vi "PH_PPPA_PowerUnit.PS Close RR.vi"(0 "i ref in":refnum<vi>, 5 "error in (no error)":errorcluster) -> (14 "i ref out":refnum<vi>, 19 "error out":errorcluster)   [LabVIEW 2014, in "PH_PPPA_PowerUnit.lvlib"]
uses:
  PH_PPPA_PowerUnit.lvlib
  PH_Beckhoff_PP_PU/PH_Beckhoff_PP_PU.lvlib
  PH_PowerUnit_BaseClass/PH_PowerUnit_BaseClass.lvlib
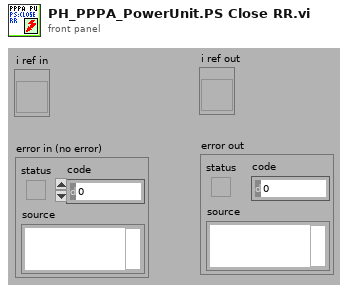
[diagram p1: front panel]
types:
  T1 = typedef "PH_PPPA_PowerUnit.lvlib/PH_PPPA_PowerUnit.i attribute.ctl" = cluster{"GUI Refs":cluster{"Ignitron":refnum<vi>, "Rossrelais":refnum<vi>, "Set Voltage":refnum<vi>, "PSU":refnum<vi>, "EOC":refnum<vi>, "Trigger":refnum<vi>}, "Ignitron":T2, "PSU":T4, "Dump Ross Relais":T5, "Trigger":cluster{"State Device":T3, "linked?":bool}, "Timing Settings":cluster{"Prdc Fast?":bool, "Default Value Periodic Interval":i32, "Mercury on since":dbl, "Warm up Time Mercury [s]":dbl}, "Set Voltage [V]":dbl, "19er Ignitionbox":string}
  T2 = typedef "PH_PP_Common.lvlib/PH_PP_Common.Ignitron Attributes.ctl" = cluster{"State Device":T3, "linked?":bool}
  T3 = typedef "PH_StatusHandler.lvlib/PH_StatusHandler.Status.ctl" = i16
  T4 = typedef "PH_PP_Common.lvlib/PH_PP_Common.PSU Attributes.ctl" = cluster{"lower limit [V]":dbl, "upper limit [V]":dbl, "Voltage set":bool, "State Device":T3, "linked?":bool}
  T5 = typedef "PH_PP_Common.lvlib/PH_PP_Common.Ross Relais Attributes.ctl" = cluster{"State Device":T3, "linked?":bool}
  T6 = typedef "PH_PowerUnit_BaseClass.lvlib/PH_PowerUnit_BaseClass.i attribute.ctl" = cluster{"Constructor finished":bool, "PU":cluster{"In use":bool, "Service ID in use":i32, "GUI Ref":refnum<vi>}, "Enabling":cluster{"State":T7, "GUI Ref":refnum<vi>}, "Timing":cluster{"Last Shot":dbl, "Time between Shots [Sec]":dbl, "Waiting Time over?":bool, "Service ID Waiting Time":i32, "GUI Ref":refnum<vi>, "Instance":cluster{"Status":T3, "linked?":bool, "GUI Ref":refnum<vi>}}, "Sequencer":cluster{"SM State":string, "GUI Ref":refnum<vi>, "linked":bool}, "Subscribed Trendmssgs":cluster{"Tagname":string, "Status":T3, "linked?":bool, "Shot Condition":T3, "GUI Ref":refnum<vi>}[], "PP PU":T8, "Default Voltage (V)":dbl, "GUI Refs":T9, "PSDB data":cluster{"Shot Voltage [V]":dbl, "State TO SM":T10, "Write 2 early":bool}, "State TO SM":T10}
  T7 = typedef "PH_SystemInformation.lvlib/PH_SystemInformationEnabling State.ctl" = i32
  T8 = typedef "PH_PP_Common.lvlib/PH_PP_Common.PUs.ctl" = enum16{"no Info", "PA-19mm-1", "PA-19mm-2", "PA-45mm-PILC", "PA-45mm-MAIN", "MA-PU-1", "MA-PU-2", "MA-PU-3", "MA-PU-4", "MA-PU-5", "MA-PU-6", "MA-FR", "MA-PILC", "PA-45mm-DP"}
  T9 = typedef "PH_PowerUnit_BaseClass.lvlib/PH_PowerUnit_BaseClass.GUI Refs.ctl" = cluster{"Delete Inst":refnum<vi>, "State TO SM":refnum<vi>, "State SM":refnum<vi>, "Fire":refnum<vi>}
  T10 = typedef "PH_PowerUnit_BaseClass.lvlib/PH_PowerUnit_BaseClass.SM States.ctl" = enum16{".", "Stand by", "Switch PU on", "Configure", "Set Default Voltage", "Set STANDBY", "Set READY", "Wait for Shot Cmd", "Open Dump Rods", "Open Ross Relais", "Close Ross Relais", "Switch PSU on", "Switch PSU off", "Charge", "Switch GD Channel on", "Close Dump Rods", "Rods-TO", "RR-TO", "PSU-TO", "Trigger-TO"}
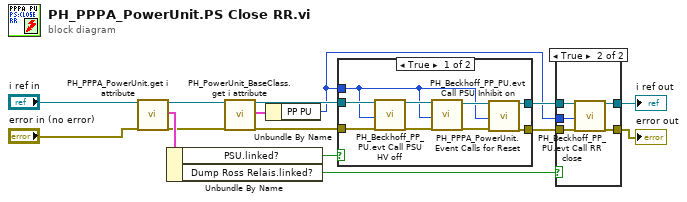
[diagram p0: block diagram]
diagram:
  n1 = call "PH_PPPA_PowerUnit.get i attribute.vi"("i ref in"="i ref in", "error in (no error)"="error in (no error)") -> ("i ref out"=w2:refnum<vi>, "i attribute"=w13:T1, "error out"=w1:errorcluster)  [unwired: 15 in]
  n2 = Unbundle By Name(w13) -> ("PSU.linked?"=w9:bool, "Dump Ross Relais.linked?"=w12:bool)
  n3 = call "PH_PowerUnit_BaseClass.get i attribute.vi"("i ref in"=w2, "error in (no error)"=w1) -> ("i ref out"=w5:refnum<vi>, "i attribute"=w4:T6, "error out"=w6:errorcluster)  [unwired: 15 in]
  n4 = Unbundle By Name(w4) -> ("PP PU"=w3:T8)
  n5 = case shown="True" w9 {
    tunnel: w5 -> [w23 w26]
    tunnel: w6 -> [w21 w25]
    tunnel: [w19 w26] -> w7
    tunnel: [w17 w25] -> w8
    tunnel: w3 -> [w16 _]
    frame True {
      n6 = call "PH_Beckhoff_PP_PU.evt Call PSU HV off.vi"("i ref in"=w23, "PU"=w16, "error in"=w21) -> ("i ref out"=w22:refnum<vi>, "error out"=w20:errorcluster)  [unwired: 15 in]
      n7 = call "PH_Beckhoff_PP_PU.evt Call PSU Inhibit on.vi"("i ref in"=w22, "PU"=w16, "error in"=w20) -> ("i ref out"=w24:refnum<vi>, "error out"=w18:errorcluster)  [unwired: 15 in]
      n8 = call "PH_PPPA_PowerUnit.Event Calls for Reset.vi"("i ref in"=w24, "PU"=w16, "error in (no error)"=w18) -> ("i ref out"=w19:refnum<vi>, "error out"=w17:errorcluster)  [unwired: 15 in]
    }
    frame False {
    }
  }
  n9 = case shown="True" w12 {
    tunnel: w7 -> [w28 w33]
    tunnel: w8 -> [w27 w32]
    tunnel: [w28 w31] -> w11
    tunnel: [w27 w30] -> w10
    tunnel: w3 -> [_ w29]
    frame False {
    }
    frame True {
      n10 = call "PH_Beckhoff_PP_PU.evt Call RR close.vi"("i ref in"=w33, "PU"=w29, "error in"=w32) -> ("i ref out"=w31:refnum<vi>, "error out"=w30:errorcluster)  [unwired: 15 in]
    }
  }
  "error out" <- w10
  "i ref out" <- w11
